vi "Generate External Sensors Table.vi"(9 "External Sensor Names":string[](array[string]), 11 "WithOffset":bool) -> (2 "External Sensors":cluster{"Name":string, "Value":dbl}[](array[cluster]))   [LabVIEW 2009]
uses:
  Global Data/Cartesian Measurment Actions.ctl
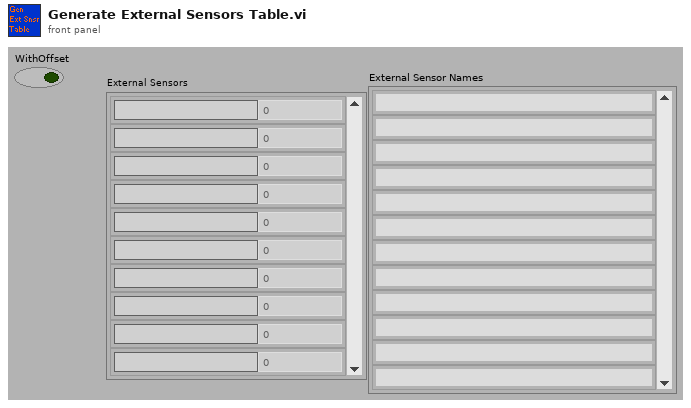
[diagram p1: front panel]
types:
  T1 = typedef "Cartesian Measurment Actions.ctl" = enum16{"Set Data", "Get", "Init", "Set Offsets"}
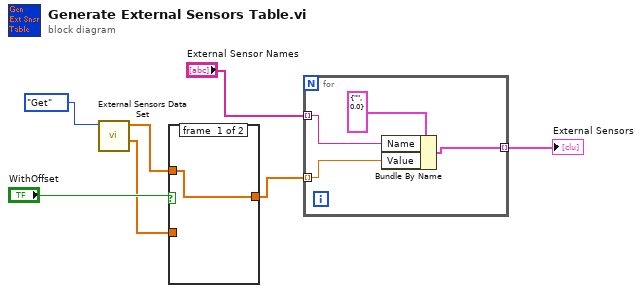
[diagram p0: block diagram]
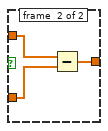
[diagram p2: hidden frame]
diagram:
  n1 = call "External Sensors Data Set.vi"("Measurement Actions"=Cartesian_Measurment_Actions."Get") -> ("Offsets"=w3:dbl[], "External Sensors Out"=w2:dbl[])  [unwired: 3 in, 6 out]
  n2 = case shown="False" "WithOffset" {
    tunnel: w3 -> [_ w10]
    tunnel: w2 -> [w8 w11]
    tunnel: [w8 w9] -> w1
    frame #0 {
    }
    frame #1 {
      n3 = Subtract(x=w11, y=w10) -> (x-y=w9:dbl[])
    }
  }
  n4 = for {
    tunnel: w1 -> [w14] mode=indexing
    tunnel: "External Sensor Names" -> [w13] mode=indexing
    tunnel: [w12] -> w7 mode=indexing
    n5 = Bundle By Name(cluster=cluster{"Name":string, "Value":dbl} {"Name"="", "Value"=0.0} ("Cluster"), "Name"=w13, "Value"=w14) -> (w12:cluster{"Name":string, "Value":dbl})
  }
  "External Sensors" <- w7
